vi "SPADQ_Init.vi"(8 "error in":errorcluster, 10 "adq_num":i32=1) -> (0 "error out":errorcluster, 1 "Info":T1, 2 "adq_cu_ptr":refnum<k24>, 3 "ADQAPI Ref":refnum<k24>)   [LabVIEW 2022 SP3]
uses:
  C:/Windows/System32/ADQAPI_dotNet_helper.dll
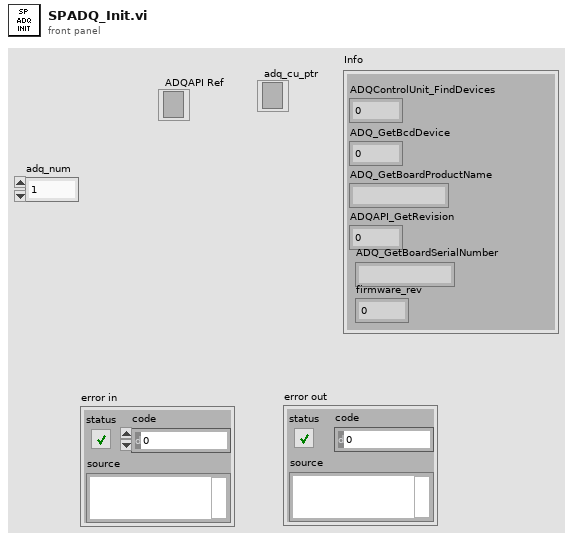
[diagram p1: front panel]
types:
  T1 = cluster{"ADQControlUnit_FindDevices":i32, "ADQ_GetBcdDevice":u32, "ADQ_GetBoardProductName":string, "ADQAPI_GetRevision":i32, "ADQ_GetBoardSerialNumber":string, "firmware_rev":i32}
  T2 = cluster{"ADQControlUnit_FindDevices":i32, "ADQ_GetBcdDevice":u32, "ADQ_GetBoardProductName":string, "ADQAPI_GetRevision":i32, "ADQ_GetBoardSerialNumber":string, "int_p_value":i32}
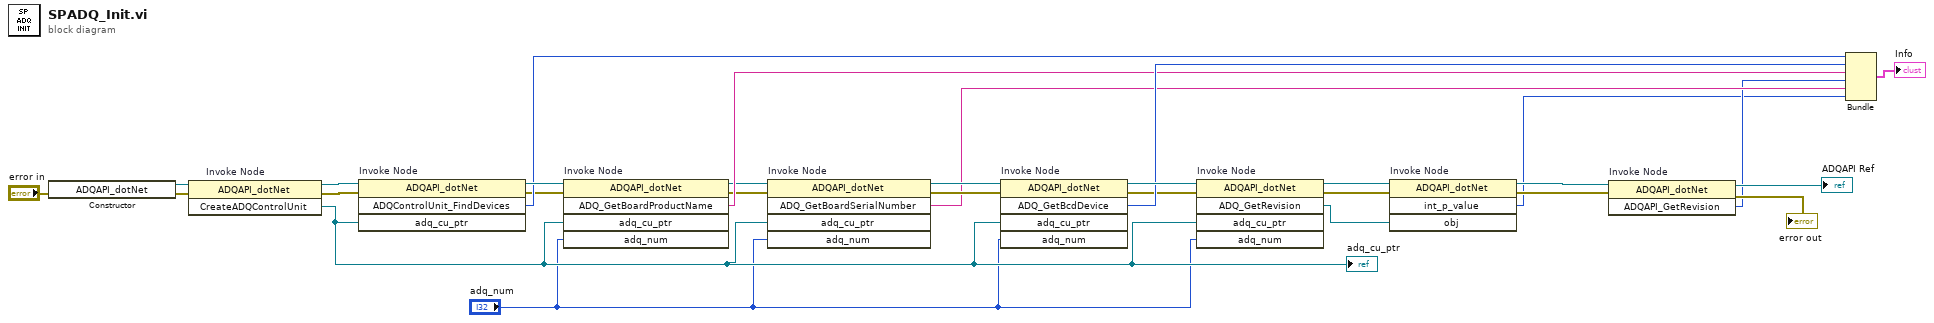
[diagram p0: block diagram]
diagram:
  n1 = constructor class="ADQAPI_dotNet"(error in="error in") -> (reference out=w18:refnum<k24>, error out=w28:errorcluster)  [unwired: 2 in, 1 out]
  n2 = invoke on="Invoke Node" class="ADQAPI_dotNet" method="CreateADQControlUnit"(reference=w18, error in=w28) -> (reference out=w29:refnum<k24>, error out=w27:errorcluster, "CreateADQControlUnit"=w2:refnum<k24>)  [unwired: 1 in]
  "adq_cu_ptr" <- w2
  n3 = invoke on="Invoke Node" class="ADQAPI_dotNet" method="ADQControlUnit_FindDevices"(reference=w29, error in=w27, "adq_cu_ptr"=w2) -> (reference out=w26:refnum<k24>, error out=w7:errorcluster, "ADQControlUnit_FindDevices"=w22:i32)  [unwired: 1 in, 1 out]
  n4 = invoke on="Invoke Node" class="ADQAPI_dotNet" method="ADQ_GetBoardProductName"(reference=w26, error in=w7, "adq_cu_ptr"=w2, "adq_num"="adq_num") -> (reference out=w12:refnum<k24>, error out=w8:errorcluster, "ADQ_GetBoardProductName"=w20:string)  [unwired: 1 in, 2 out]
  n5 = invoke on="Invoke Node" class="ADQAPI_dotNet" method="ADQ_GetBoardSerialNumber"(reference=w12, error in=w8, "adq_cu_ptr"=w2, "adq_num"="adq_num") -> (reference out=w9:refnum<k24>, error out=w10:errorcluster, "ADQ_GetBoardSerialNumber"=w6:string)  [unwired: 1 in, 2 out]
  n6 = invoke on="Invoke Node" class="ADQAPI_dotNet" method="ADQ_GetBcdDevice"(reference=w9, error in=w10, "adq_cu_ptr"=w2, "adq_num"="adq_num") -> (reference out=w25:refnum<k24>, error out=w11:errorcluster, "ADQ_GetBcdDevice"=w21:u32)  [unwired: 1 in, 2 out]
  n7 = invoke on="Invoke Node" class="ADQAPI_dotNet" method="ADQ_GetRevision"(reference=w25, error in=w11, "adq_cu_ptr"=w2, "adq_num"="adq_num") -> (reference out=w17:refnum<k24>, error out=w15:errorcluster, "ADQ_GetRevision"=w13:refnum<k24>)  [unwired: 1 in, 2 out]
  n8 = invoke on="Invoke Node" class="ADQAPI_dotNet" method="int_p_value"(reference=w17, error in=w15, "obj"=w13) -> (reference out=w16:refnum<k24>, error out=w14:errorcluster, "int_p_value"=w4:i32)  [unwired: 1 in, 1 out]
  n9 = invoke on="Invoke Node" class="ADQAPI_dotNet" method="ADQAPI_GetRevision"(reference=w16, error in=w14) -> (reference out=→"ADQAPI Ref":refnum<k24>, error out=→"error out":errorcluster, "ADQAPI_GetRevision"=w5:i32)  [unwired: 1 in]
  n10 = Bundle("ADQControlUnit_FindDevices"=w22, "ADQ_GetBcdDevice"=w21, "ADQ_GetBoardProductName"=w20, "ADQAPI_GetRevision"=w5, "ADQ_GetBoardSerialNumber"=w6, "int_p_value"=w4) -> (→"Info":T2)  [unwired: 1 in]
